vi "tcp_client.vi"() -> ()   [LabVIEW 2019]
panel:
  in  "stop_query 3":bool
  out "spill_id 3":i32
  out "client_step 3":i32
  out "BOS 3":bool=TRUE
  out "EOS 3":bool=TRUE
  out "status 3":bool
  in  "stop_query 2":bool
  out "spill_id 2":i32
  out "client_step 2":i32
  out "BOS 2":bool=TRUE
  out "EOS 2":bool=TRUE
  out "status 2":bool
  out "status":bool
  out "EOS":bool=TRUE
  out "BOS":bool=TRUE
  out "client_step":i32
  in  "stop_query":bool
  out "spill_id":i32
  # "ASAP Mode #2"
  # "ASAP Mode"
  # "BOS Mode"
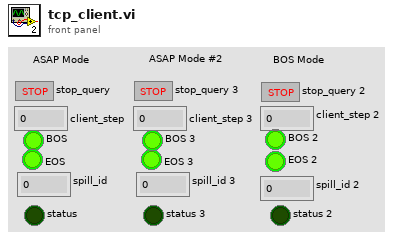
[diagram p1: front panel]
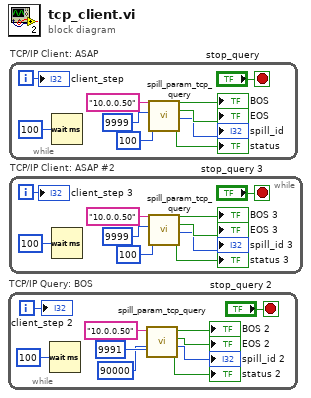
[diagram p0: block diagram]
diagram:
  n1 = while "TCP/IP Query: BOS" {
    i -> [w1]
    stop <- "stop_query 2" stop-if-true
    n2 = Wait (ms)(milliseconds to wait=u32 100) -> ()  [unwired: 1 out]
    n3 = call "spill_param_tcp_query.vi"("wait_time"=90000, "port"=u16 9991, "address"="10.0.0.50") -> ("status"=→"status 2":bool, "spill_id"=→"spill_id 2":i32, "EOS"=→"EOS 2":bool, "BOS"=→"BOS 2":bool)  [unwired: 3 in]
    "client_step 2" <- w1
  }
  n4 = while "TCP/IP Client: ASAP" {
    i -> [w11]
    stop <- "stop_query" stop-if-true
    n5 = Wait (ms)(milliseconds to wait=u32 100) -> ()  [unwired: 1 out]
    n6 = call "spill_param_tcp_query.vi"("wait_time"=100, "port"=u16 9999, "address"="10.0.0.50") -> ("status"=→"status":bool, "spill_id"=→"spill_id":i32, "EOS"=→"EOS":bool, "BOS"=→"BOS":bool)  [unwired: 3 in]
    "client_step" <- w11
  }
  n7 = while "TCP/IP Client: ASAP #2" {
    i -> [w21]
    stop <- "stop_query 3" stop-if-true
    n8 = Wait (ms)(milliseconds to wait=u32 100) -> ()  [unwired: 1 out]
    n9 = call "spill_param_tcp_query.vi"("wait_time"=100, "port"=u16 9999, "address"="10.0.0.50") -> ("status"=→"status 3":bool, "spill_id"=→"spill_id 3":i32, "EOS"=→"EOS 3":bool, "BOS"=→"BOS 3":bool)  [unwired: 3 in]
    "client_step 3" <- w21
  }
